vi "Serial_Port_Select.vi"(8 "error in":errorcluster, 11 "PortString":string) -> (0 "error out":errorcluster, 2 "SelectedPort":string, 3 "PortList":string[](array[string]))   [LabVIEW 2016]
uses:
  <vilib>/Instr/_visa.llb/VISA Find Search Mode.ctl
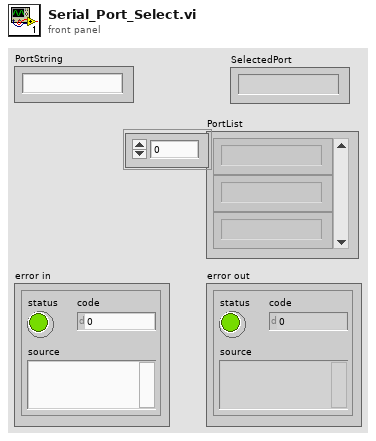
[diagram p1: front panel]
types:
  T1 = typedef "VISA Find Search Mode.ctl" = u32
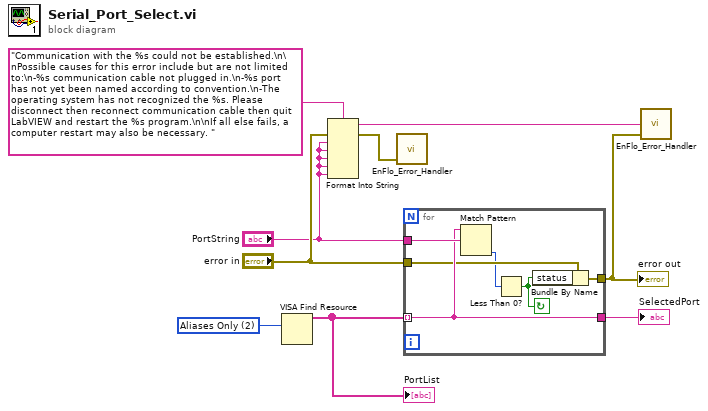
[diagram p0: block diagram]
diagram:
  w9 = T1 2 items=["Canonical Names Only"=0, "Aliases Only"=2, "Include Matching Aliases"=3, "Include All Aliases"=4] ("Search Mode")
  n1 = VISA Find Resource(10:w9) -> (3:w8:string[])  [unwired: 1 in, 3 out]
  "PortList" <- w8
  n2 = Format Into String(format string="Communication with the %s could not be established.\n\nPossible causes for this error include but are not limited to:\n-%s communication cable not plugged in.\n-%s port has not yet been named according to convention.\n-The operating system has not recognized the %s. Please disconnect then reconnect communication cable then quit LabVIEW and restart the %s program.\n\nIf all else fails, a computer restart may also be necessary. " ("string"), error in="error in", "PortString", "PortString", "PortString", "PortString", "PortString") -> (resulting string=w4:string, error out=w2:errorcluster)  [unwired: 1 in]
  n3 = call "EnFlo_Error_Handler.vi"("error in (no error)"=w2) -> ()  [unwired: 2 in, 3 out]
  n4 = for {
    tunnel: w8 -> [w14] mode=indexing
    tunnel: "PortString" -> [w15]
    tunnel: [w14] -> w7
    tunnel: "error in" -> [w13]
    tunnel: [w10] -> w6
    stop <- w11 continue-if-true
    n5 = Match Pattern(string=w14, regular expression=w15) -> (offset past match=w12:i32)  [unwired: 4 out]
    n6 = Less Than 0?(x=w12) -> (x < 0?=w11:bool)
    n7 = Bundle By Name(cluster=w13, "status"=w11) -> (w10:errorcluster)
  }
  "SelectedPort" <- w7
  "error out" <- w6
  n8 = call "EnFlo_Error_Handler.vi"("error in (no error)"=w6, "Error Type"=w4) -> ()  [unwired: 1 in, 3 out]
